vi "zadanie_2.vi"() -> ()   [LabVIEW 2020]
panel:
  in  "Wylacz program":bool
  in  "Wybierz opoznienie wykonania petli For":u16(ring) items=["500 ms", "250 ms", "100 ms"]
  out "Ilosc wykonan liczby For":i32
  in  "Wprowadz liczbe wykonan petli For":i32
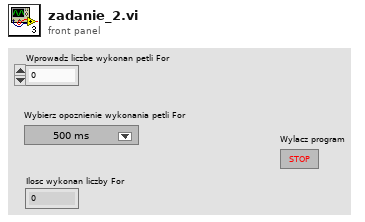
[diagram p1: front panel]
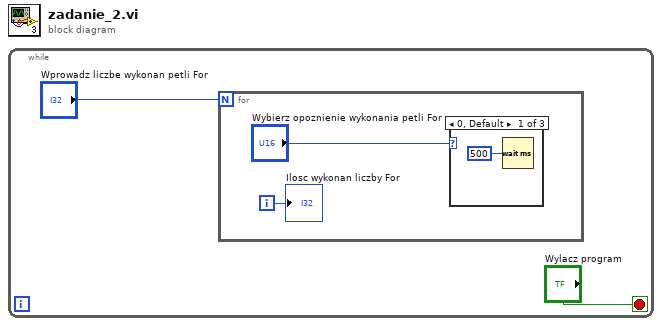
[diagram p0: block diagram]
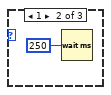
[diagram p2: hidden frame]
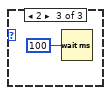
[diagram p3: hidden frame]
diagram:
  n1 = while {
    stop <- "Wylacz program" stop-if-true
    n2 = for {
      N: "Wprowadz liczbe wykonan petli For" -> [_]
      i -> [w4]
      n3 = case shown="0, Default" "Wybierz opoznienie wykonania petli For" {
        frame 0, Default {
          n4 = Wait (ms)(milliseconds to wait=u32 500) -> ()  [unwired: 1 out]
        }
        frame 1 {
          n5 = Wait (ms)(milliseconds to wait=u32 250) -> ()  [unwired: 1 out]
        }
        frame 2 {
          n6 = Wait (ms)(milliseconds to wait=u32 100) -> ()  [unwired: 1 out]
        }
      }
      "Ilosc wykonan liczby For" <- w4
    }
  }
